vi "Set Reference Trigger Attributes.vi"(0 "task in":refnum<k21>, 1 "trigger channel name":string, 5 "level trigger configuration":T1 {"hysteresis" format="%.2p"; "slope" items=["Falling", "Rising"]; "level" format="%.2p"}, 11 "error in":errorcluster, 12 "pretrigger samples":i32) -> (4 "task out":refnum<k21>, 15 "error out":errorcluster)   [LabVIEW 2024, in "Dynamic Signal Acquisition (Interactive) UI.lvlib"]
doc: "Set SV Trigger Attributes."
uses:
  <vilib>/addons/_NISVFA/_Shared subVIs/Controls/svc_Analog Level Trigger Configuration.ctl
  <vilib>/addons/Sound and Vibration/svt_DAQmx/subVIs/sv_SetCustomAttributeBoolean.vi
  <vilib>/addons/Sound and Vibration/svt_DAQmx/subVIs/sv_SetCustomAttributeDouble.vi
  <vilib>/addons/Sound and Vibration/svt_DAQmx/subVIs/sv_SetCustomAttributeInt32.vi
  Dynamic Signal Acquisition (Interactive) UI.lvlib
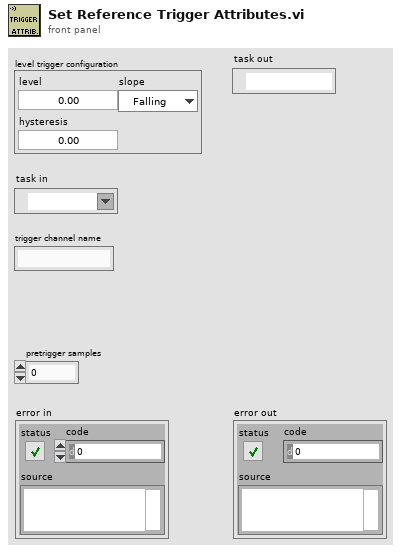
[diagram p1: front panel]
types:
  T1 = typedef "svc_Analog Level Trigger Configuration.ctl" = cluster{"level":dbl, "slope":u16, "hysteresis":dbl}
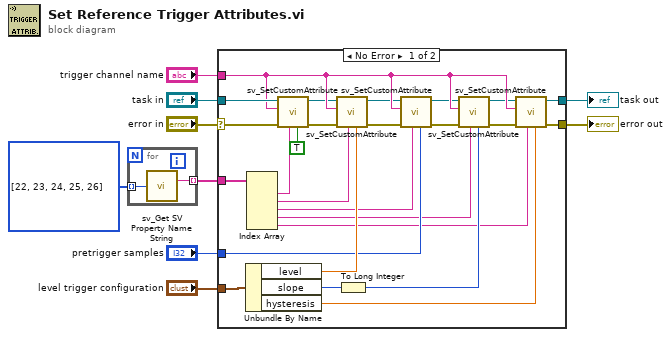
[diagram p0: block diagram]
diagram:
  w6 = u16[] [22, 23, 24, 25, 26] items=["Engineering units", "Custom unit label", "Weighting filter", "Pregain", "Octave standard", "Octave bandwidth", "Octave low band", "Octave high band", "Spectrum skewed", "Samples / revolution", "Order", "Tachometer", "Pulses Per Revolution", "Rotation Direction", "Probe Angle", "Pair", "Channel Alias", "Tachometer Threshold", "Tachometer Slope", "Max Order", "Sensor Location", "Sensor Orientation", "Analog Software Trigger", "Trigger Level", "Pretrigger Samples", "Trigger Slope", "Trigger Hysteresis"]
  n1 = for {
    tunnel: [w11] -> w1 mode=indexing
    tunnel: w6 -> [w10] mode=indexing
    n2 = call <vilib>:"sv_Get SV Property Name String.vi"("property"=w10) -> ("TDMS property name"=w11:string)  [unwired: 13 in, 1 out]
  }
  n3 = case shown="No Error" "error in" {
    selector: "error in" -> [w30 w38]
    tunnel: "level trigger configuration" -> [w34 _]
    tunnel: [w33 w38] -> w8
    tunnel: [w32 w39] -> w7
    tunnel: "pretrigger samples" -> [w29 _]
    tunnel: "task in" -> [w28 w39]
    tunnel: "trigger channel name" -> [w27 _]
    tunnel: w1 -> [w12 _]
    frame No Error {
      n4 = Unbundle By Name(w34) -> ("level"=w37:dbl, "slope"=w36:u16, "hysteresis"=w35:dbl)
      n5 = Index Array(array=w12) -> (element #1=w18:string, element #2=w17:string, element #3=w16:string, element #4=w15:string, element #5=w13:string)  [unwired: 5 in]
      n6 = call-poly <vilib>:"sv_SetCustomAttribute.vi"("Attribute Value"=TRUE ("Boolean"), "Attribute Name"=w18, "error in"=w30, "Active Channel"=w27, "task in"=w28) -> ("error out"=w20:errorcluster, "task out"=w19:refnum<k21>)  [unwired: 5 in]
      n7 = call-poly <vilib>:"sv_SetCustomAttribute.vi"("Attribute Value"=w37, "Attribute Name"=w17, "error in"=w20, "Active Channel"=w27, "task/channels in"=w19) -> ("error out"=w22:errorcluster, "task out"=w21:refnum<k21>)  [unwired: 5 in]
      n8 = To Long Integer(number=w36) -> (32bit integer=w14:i32)
      n9 = call-poly <vilib>:"sv_SetCustomAttribute.vi"("Attribute Value"=w29, "Attribute Name"=w16, "error in"=w22, "Active Channel"=w27, "task/channels in"=w21) -> ("error out"=w23:errorcluster, "task out"=w24:refnum<k21>)  [unwired: 5 in]
      n10 = call-poly <vilib>:"sv_SetCustomAttribute.vi"("Attribute Value"=w14, "Attribute Name"=w15, "error in"=w23, "Active Channel"=w27, "task/channels in"=w24) -> ("error out"=w25:errorcluster, "task out"=w26:refnum<k21>)  [unwired: 5 in]
      n11 = call-poly <vilib>:"sv_SetCustomAttribute.vi"("Attribute Value"=w35, "Attribute Name"=w13, "error in"=w25, "Active Channel"=w27, "task/channels in"=w26) -> ("error out"=w33:errorcluster, "task out"=w32:refnum<k21>)  [unwired: 5 in]
    }
    frame Error {
    }
  }
  "error out" <- w8
  "task out" <- w7
